vi "Write DS402 Drive VARs.vi"(7 "R/W Case":T7, 8 "error in (no error)":errorcluster, 9 "Input FIFO buffer in":dbl[](array[numeric]), 10 "I/O Output Data In":T1 {"BD Refs"."Data Reference" format="%.0x"}, 11 "I/O Output Vars in":T4[](array[typedef]) {"VS ref" format="%.0x"}) -> (0 "error out":errorcluster, 1 "Input FIFO buffer out":dbl[](array[numeric]), 2 "I/O Output Data Out":T1 {"BD Refs"."Data Reference" format="%.0x"}, 3 "I/O Output Vars out":T4[](array[typedef]) {"VS ref" format="%.0x"})   [LabVIEW 2016, in "Scan Engine Custom Device.lvlib"]
uses:
  Scan Engine Custom Device.lvlib
  Type Defs/RW Case.ctl
  Type Defs/DS402 Drive ECAT Slave IOV Cluster.ctl
  <vilib>/NI Veristand/Custom Device API/Custom Device Item Ref.ctl
  Type Defs/UDV Data Type.ctl
  Type Defs/Output Data.ctl
  <vilib>/NI Veristand/Custom Device API/Block Data Reference.ctl
  <vilib>/NI Veristand/Custom Device API/Data Reference.ctl
  <vilib>/NI Veristand/Custom Device API/Global Data Refs.vi
  <vilib>/NI Veristand/Custom Device API/Custom Device API.lvlib
  <vilib>/NI Veristand/Custom Device Tools/Custom Device Utility Library/Custom Device Utility Library.lvlib
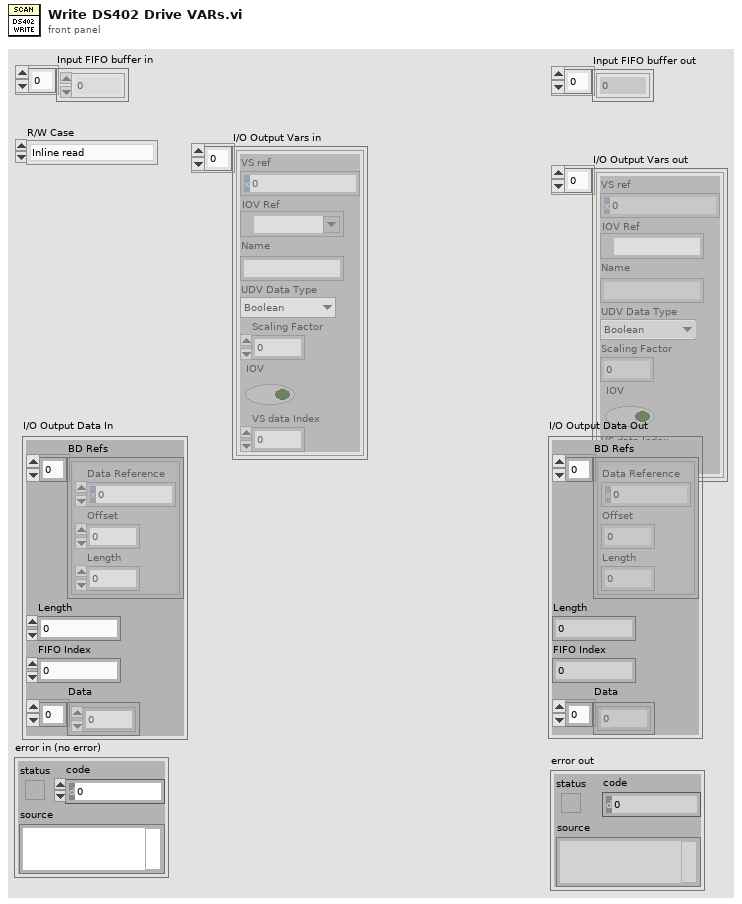
[diagram p1: front panel]
types:
  T1 = typedef "Scan Engine Custom Device.lvlib/Output Data.ctl" = cluster{"BD Refs":T2[], "Length":i32, "FIFO Index":i32, "Data":dbl[]}
  T2 = typedef "Custom Device API.lvlib/Block Data Reference.ctl" = cluster{"Data Reference":T3, "Offset":u64, "Length":u64}
  T3 = typedef "Custom Device API.lvlib/Data Reference.ctl" = i32
  T4 = typedef "Scan Engine Custom Device.lvlib/DS402 Drive ECAT Slave IOV Cluster.ctl" = cluster{"VS ref":T5, "IOV Ref":refnum<k21>, "Name":string, "UDV Data Type":T6, "Scaling Factor":dbl, "IOV":bool, "VS data Index":i32}
  T5 = typedef "Custom Device API.lvlib/Custom Device Item Ref.ctl" = u64
  T6 = typedef "Scan Engine Custom Device.lvlib/UDV Data Type.ctl" = enum16{"Boolean", "Fixed Point", "Int8", "Int16", "Int32", "Int64", "U32 Bit Field", "UInt8", "UInt16", "UInt32", "UInt64", "Other"}
  T7 = typedef "Scan Engine Custom Device.lvlib/RW Case.ctl" = enum16{"Inline read", "Inline write", "Async - Inline loop read", "Async - Inline loop write", "Async loop (read/write)"}
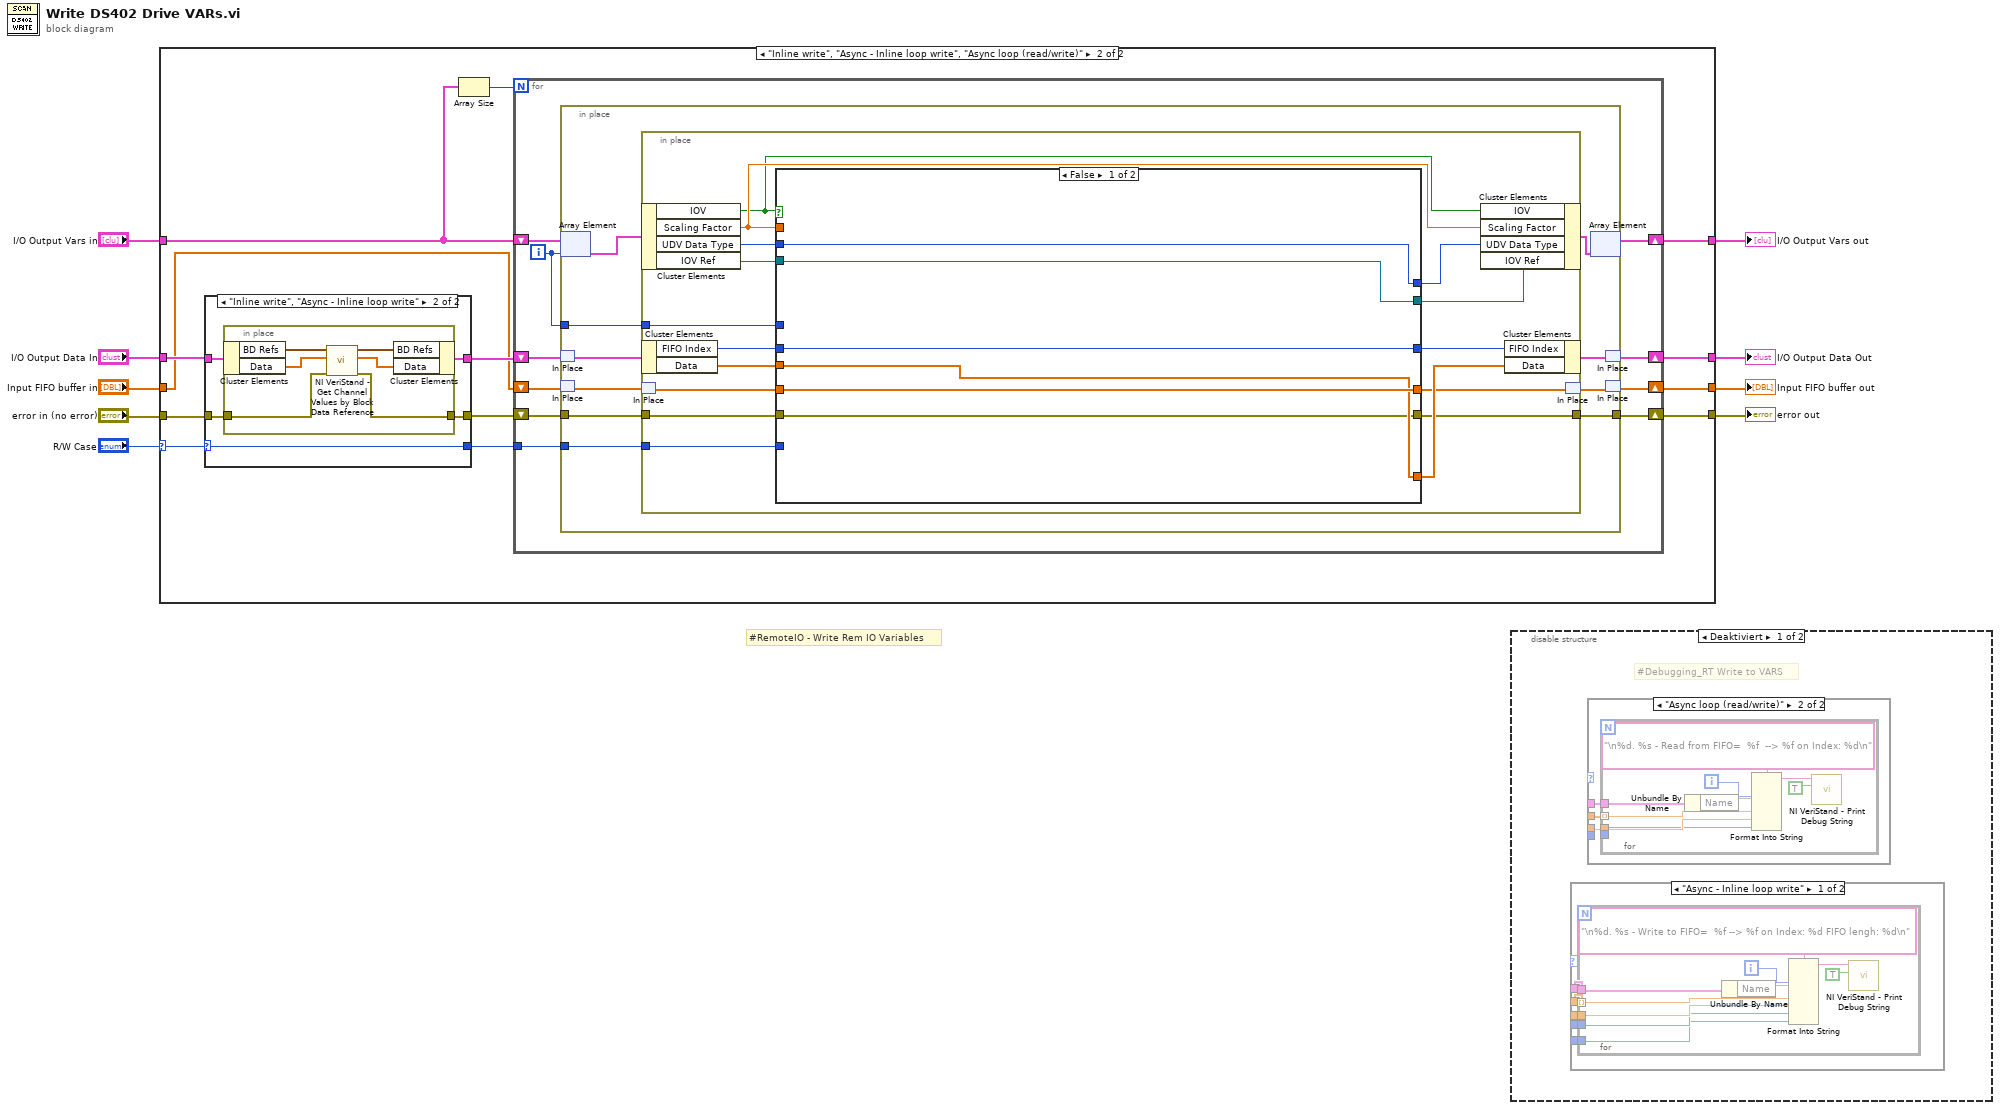
[diagram p0: block diagram]
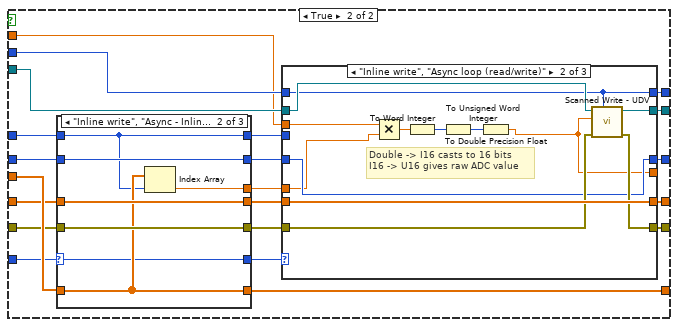
[diagram p3: hidden frame]
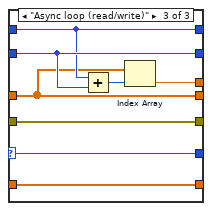
[diagram p5: hidden frame]
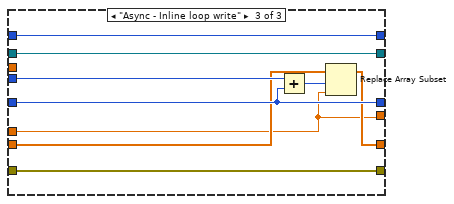
[diagram p7: hidden frame]
diagram:
  # "#RemoteIO - Write Rem IO Variables"
  n1 = case shown="\"Inline write\", \"Async - Inline loop write\", \"Async loop (read/write)\"" "R/W Case" {
    selector: "R/W Case" -> [_ w22]
    tunnel: [w11 w26] -> w5
    tunnel: "Input FIFO buffer in" -> [w11 w14]
    tunnel: [w12 w16] -> w2
    tunnel: [w13 w25] -> w6
    tunnel: "I/O Output Data In" -> [w12 w20]
    tunnel: "I/O Output Vars in" -> [w13 w24]
    tunnel: [w10 w15] -> w4
    tunnel: "error in (no error)" -> [w10 w21]
    frame Default {
    }
    frame "Inline write", "Async - Inline loop write", "Async loop (read/write)" {
      n2 = case shown="\"Inline write\", \"Async - Inline loop write\"" w22 {
        selector: w22 -> [w139 w142]
        tunnel: w20 -> [w140 w146]
        tunnel: w21 -> [w141 w145]
        tunnel: [w141 w144] -> w18
        tunnel: [w140 w143] -> w19
        tunnel: [w139 w142] -> w17
        frame Default {
        }
        frame "Inline write", "Async - Inline loop write" {
          n3 = in-place {
            in-place-border: w145 -> [w148]
            in-place-border: [w147] -> w144
            n4 = in-place-cluster #1(w146) -> ("BD Refs"=w152:T2[], "Data"=w150:dbl[])
            n5 = call <vilib>:"NI VeriStand - Get Channel Values by Block Data Reference.vi"("error in (no error)"=w148, "Values Array in"=w150, "Block Data Ref"=w152) -> ("error out"=w147:errorcluster, "Values Array out"=w149:dbl[], "Block Data Ref dup"=w151:T2[])  [unwired: 6 in]
            n6 = in-place-cluster #1("BD Refs"=w151, "Data"=w149) -> (w143:T1)
          }
        }
      }
      n7 = Array Size(array=w24) -> (size(s)=w23:i32)
      n8 = for {
        N: w23 -> [_]
        shift-right: [w35] -> w25
        shift-left: w24 -> [w36]
        shift-right: [w27] -> w16
        shift-left: w19 -> [w30]
        shift-right: [w33] -> w26
        shift-left: w14 -> [w34]
        shift-right: [w31] -> w15
        shift-left: w18 -> [w32]
        tunnel: w17 -> [w29]
        i -> [w28]
        n9 = in-place {
          in-place-border: w32 -> [w44]
          in-place-border: [w38] -> w31
          in-place-border: w29 -> [w43]
          in-place-border: w28 -> [w42]
          n10 = in-place-array #2(w36, w28) -> (w37:T4)
          n11 = in-place-match #3(w30) -> (w46:T1)
          n12 = in-place-match #4(w34) -> (w45:dbl[])
          n13 = in-place {
            in-place-border: w44 -> [w50]
            in-place-border: w43 -> [w53]
            in-place-border: w42 -> [w61]
            in-place-border: [w49] -> w38
            n14 = in-place-cluster #5(w37) -> ("IOV"=w47:bool, "Scaling Factor"=w48:dbl, "UDV Data Type"=w52:T6, "IOV Ref"=w57:refnum<k21>)
            n15 = in-place-cluster #6(w46) -> ("FIFO Index"=w51:i32, "Data"=w62:dbl[])
            n16 = in-place-match #7(w45) -> (w55:dbl[])
            n17 = case shown="False" w47 {
              tunnel: w62 -> [w64 w89]
              tunnel: w61 -> [_ w88]
              tunnel: [w68 w87] -> w60
              tunnel: [w67 w86] -> w59
              tunnel: [w66 w85] -> w58
              tunnel: w57 -> [w67 w83]
              tunnel: [w64 w80] -> w56
              tunnel: w55 -> [w65 w79]
              tunnel: [w65 w78] -> w54
              tunnel: w53 -> [_ w77]
              tunnel: w52 -> [w68 w75]
              tunnel: w51 -> [w66 w74]
              tunnel: w50 -> [w63 w73]
              tunnel: [w63 w71] -> w49
              tunnel: w48 -> [_ w70]
              frame False {
              }
              frame True {
                n18 = case shown="\"Inline write\", \"Async - Inline loop write\"" w77 {
                  selector: w77 -> [w92 w97 w106]
                  tunnel: w88 -> [w90 w98 w107]
                  tunnel: w74 -> [w95 w100 w108]
                  tunnel: w79 -> [w93 w101 w105]
                  tunnel: w73 -> [w91 w102 w110]
                  tunnel: w89 -> [w94 w99 w109]
                  tunnel: [w95 w100 w108] -> w84
                  tunnel: [w94 w99 w109] -> w80
                  tunnel: [w91 w102 w110] -> w72
                  tunnel: [w93 w101 w105] -> w76
                  tunnel: [w92 w97 w106] -> w82
                  tunnel: [_ w96 w104] -> w69
                  tunnel: [w90 w98 w107] -> w81
                  frame Default {
                  }
                  frame "Inline write", "Async - Inline loop write" {
                    n19 = Index Array(array=w99, index=w98) -> (element=w96:dbl)
                  }
                  frame "Async loop (read/write)" {
                    n20 = Add(x=w107, y=w108) -> (x+y=w103:i32)
                    n21 = Index Array(array=w105, index=w103) -> (element=w104:dbl)
                  }
                }
                n22 = case shown="\"Inline write\", \"Async loop (read/write)\"" w82 {
                  tunnel: w75 -> [w112 w120 w138]
                  tunnel: w83 -> [w113 w122 w133]
                  tunnel: w84 -> [w114 w125 w135]
                  tunnel: w76 -> [w115 w129 w134]
                  tunnel: [w115 w129 w132] -> w78
                  tunnel: w81 -> [_ _ w136]
                  tunnel: [w114 w125 w135] -> w85
                  tunnel: [w113 w128 w133] -> w86
                  tunnel: [w112 w120 w138] -> w87
                  tunnel: w72 -> [w116 w127 w137]
                  tunnel: [w116 w126 w137] -> w71
                  tunnel: w69 -> [w111 w123 w130]
                  tunnel: w70 -> [_ w124 _]
                  tunnel: [w111 w121 w130] -> _
                  frame Default {
                  }
                  frame "Inline write", "Async loop (read/write)" {
                    # "Double -> I16 casts to 16 bits\nI16 -> U16 gives raw ADC value"
                    n23 = Multiply(x=w124, y=w123) -> (x*y=w119:dbl)
                    n24 = To Word Integer(number=w119) -> (16bit integer=w118:i16)
                    n25 = To Unsigned Word Integer(number=w118) -> (unsigned 16bit integer=w117:u16)
                    n26 = To Double Precision Float(number=w117) -> (double precision float=w121:dbl)
                    n27 = call "Scanned Write - UDV.vi"("UDV Data Type"=w120, "error in (no error)"=w127, "data in"=w121, "IOV ref in"=w122) -> ("error out"=w126:errorcluster, "IOV ref out"=w128:refnum<k21>)  [unwired: 6 in]
                  }
                  frame "Async - Inline loop write" {
                    n28 = Add(x=w136, y=w135) -> (x+y=w131:i32)
                    n29 = Replace Array Subset(array=w134, new element=w130, index=w131) -> (w132:dbl[])
                  }
                }
              }
            }
            n30 = in-place-cluster #5("IOV"=w47, "Scaling Factor"=w48, "UDV Data Type"=w60, "IOV Ref"=w59) -> (w41:T4)
            n31 = in-place-cluster #6("FIFO Index"=w58, "Data"=w56) -> (w40:T1)
            n32 = in-place-match #7(w54) -> (w39:dbl[])
          }
          n33 = in-place-array #2(w41) -> (w35:T4[])  [unwired: 1 out]
          n34 = in-place-match #3(w40) -> (w27:T1)
          n35 = in-place-match #4(w39) -> (w33:dbl[])
        }
      }
    }
  }
  "Input FIFO buffer out" <- w5
  "error out" <- w4
  "I/O Output Vars out" <- w6
  "I/O Output Data Out" <- w2
  n36 = disable-structure shown="Deaktiviert" {
    frame Disabled {
      # "#Debugging_RT Write to VARS"
      n37 = case shown="\"Async - Inline loop write\"" {
        selector: _ -> [_ _]
        tunnel: _ -> [w170 _]
        tunnel: _ -> [w169 _]
        tunnel: _ -> [w168 _]
        tunnel: _ -> [w167 _]
        tunnel: _ -> [w166 _]
        frame "Async - Inline loop write" {
          n38 = for {
            tunnel: w170 -> [w176]
            tunnel: w169 -> [w175] mode=indexing
            tunnel: w168 -> [w173]
            tunnel: w167 -> [w172]
            tunnel: w166 -> [w171]
            i -> [w178]
            n39 = Unbundle By Name(w176) -> ("Name"=w177)
            n40 = Format Into String(format string="\n%d. %s - Write to FIFO=  %f --> %f on Index: %d FIFO lengh: %d\n" ("Format-String"), w178, w177, w175, w173, w172, w171) -> (resulting string=w179:string)  [unwired: 2 in, 1 out]
            n41 = call <vilib>:"NI VeriStand - Print Debug String.vi"("Add to log file? (T)"=TRUE, "Message"=w179) -> ()  [unwired: 9 in, 1 out]
          }
        }
        frame Default {
        }
      }
      n42 = case shown="\"Async loop (read/write)\"" {
        selector: _ -> [_ _]
        tunnel: _ -> [_ w156]
        tunnel: _ -> [_ w155]
        tunnel: _ -> [_ w154]
        tunnel: _ -> [_ w153]
        frame "Async - Inline loop write", Default {
        }
        frame "Async loop (read/write)" {
          n43 = for {
            tunnel: w156 -> [w160]
            tunnel: w155 -> [w159] mode=indexing
            tunnel: w154 -> [w158]
            tunnel: w153 -> [w157]
            i -> [w162]
            n44 = Unbundle By Name(w160) -> ("Name"=w161)
            n45 = Format Into String(format string="\n%d. %s - Read from FIFO=  %f  --> %f on Index: %d\n" ("Format-String"), w162, w161, w159, w158, w157) -> (resulting string=w163:string)  [unwired: 2 in, 1 out]
            n46 = call <vilib>:"NI VeriStand - Print Debug String.vi"("Add to log file? (T)"=TRUE, "Message"=w163) -> ()  [unwired: 9 in, 1 out]
          }
        }
      }
    }
    frame Enabled {
    }
  }
